vi "A33ConfigureWFM_py.vi"(4 "Frequency/BW/BitRate (1000.0 Hz)":dbl=1000.0 format="%#_12g", 5 "Phase (0 deg)":dbl format="%#_12g", 6 "DC Offset (0.0 Volts)":dbl step=0.01 format="%#_12g", 7 "Waveform (0: Sine)":i32(ring) items=["Sine", "Square", "Pulse", "Ramp", "Noise", "DC", "PRBS", "Triangle"], 8 "error in (no error)":errorcluster, 9 "Amplitude (1.0 Vpp)":dbl=1.0 format="%#_12g", 10 "Channel (1: Channel1)":u16(ring)=1 items=["Channel1"=1, "Channel2"=2], 11 "socket in":refnum<class "zmq_socket.lvclass">) -> (0 "error out":errorcluster, 3 "socket out":refnum<class "zmq_socket.lvclass">)   [LabVIEW 2022 SP3]
doc: "Selects the waveform shape, frequency, amplitude, offset, and phase for a standard waveform."
uses:
  <vilib>/addons/zeromq/zmq_socket.lvclass
panel:
  out "Standalone":bool
  out "resulting string":string
  in  "Instrument":string="AG33600A_Gen1"
  # "-For ARB waveforms use separte vi\n-Pulse period,width,edges - separate vi\n-Noise/PRBS - seprate vi"
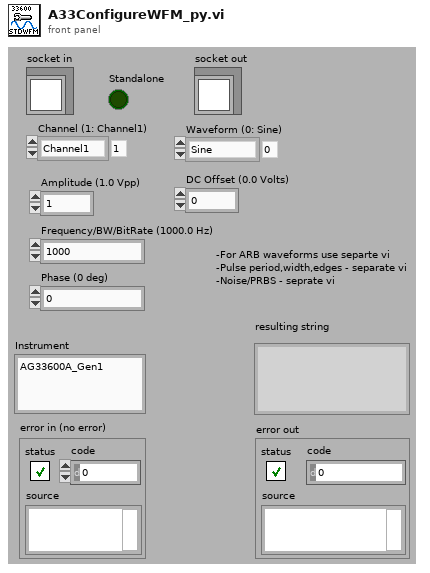
[diagram p1: front panel]
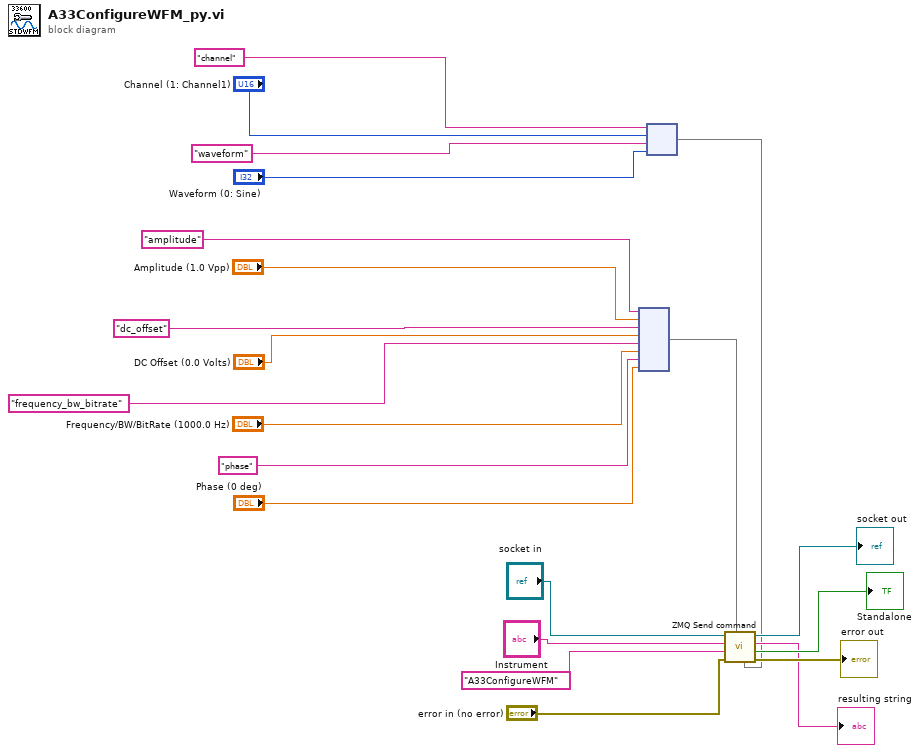
[diagram p0: block diagram]
diagram:
  n1 = node("amplitude" ("key"), "Amplitude (1.0 Vpp)", "dc_offset" ("key"), "DC Offset (0.0 Volts)", "frequency_bw_bitrate" ("key"), "Frequency/BW/BitRate (1000.0 Hz)", "phase" ("key"), "Phase (0 deg)") -> (w2:map{string, dbl})
  n2 = node("channel" ("key"), "Channel (1: Channel1)", "waveform" ("key"), "Waveform (0: Sine)") -> (w1:map{string, i32})
  n3 = call "ZMQ Send command.vi"("Int args"=w1, "DBL args"=w2, "error in"="error in (no error)", "Command"="A33ConfigureWFM", "Instrument"="Instrument", "socket in"="socket in") -> ("error out"=→"error out":errorcluster, "Standalone"=→"Standalone":bool, "Recieved message"=→"resulting string":string, "socket out"=→"socket out":refnum<class "zmq_socket.lvclass">)  [unwired: 2 in]
